vi "S2C_UNITHERM_Proc_Commands.vi"(7 "VI_Ref":refnum<vi>, 8 "Error In":errorcluster, 10 "Settings":T1, 11 "Q-Ref":refnum<queue>) -> (0 "Error Out":errorcluster, 2 "Stop?":bool, 3 "Response":variant)   [LabVIEW 2015]
uses:
  S2C_UNITHERM_Proc_Globals.vi
  _Shared/S2C_Shared_Proc_Globals.vi
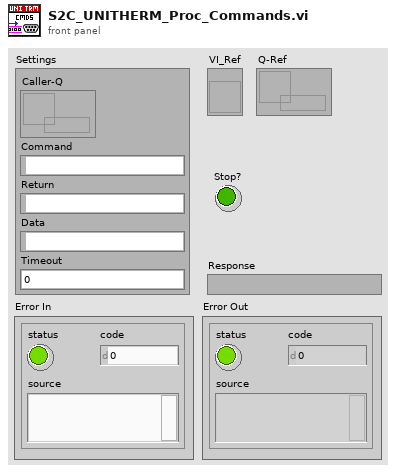
[diagram p1: front panel]
types:
  T1 = cluster{"Caller-Q":refnum<queue>, "Command":string, "Return":string, "Data":variant, "Timeout":dbl}
  T2 = enum16{"5190CR", "Fornax", "Omnia8257", "UniTherm"}
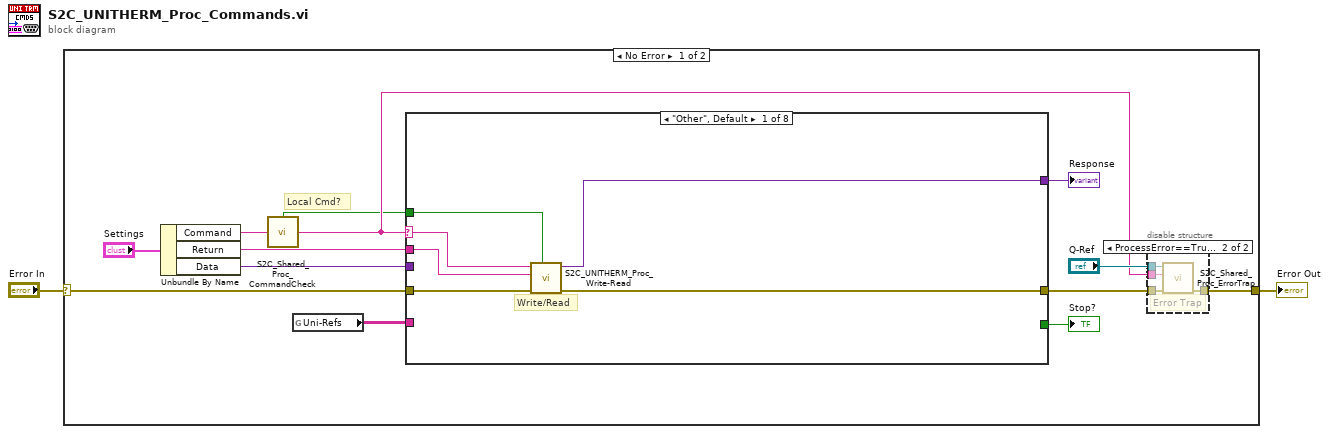
[diagram p0: block diagram]
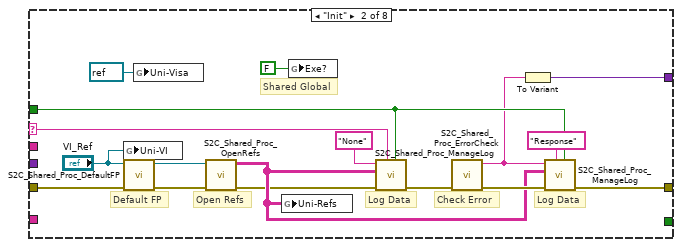
[diagram p3: hidden frame]
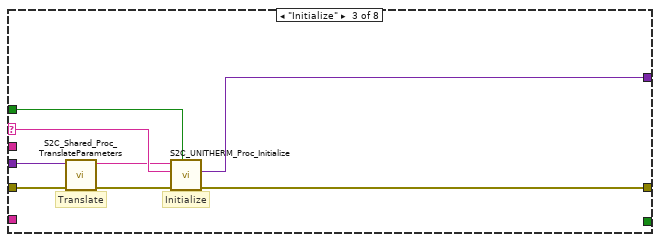
[diagram p4: hidden frame]
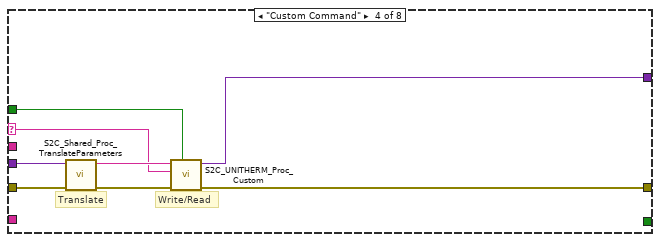
[diagram p5: hidden frame]
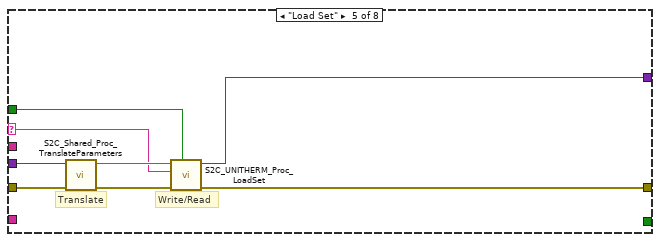
[diagram p6: hidden frame]
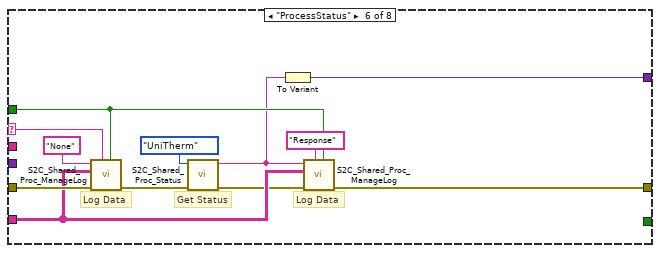
[diagram p7: hidden frame]
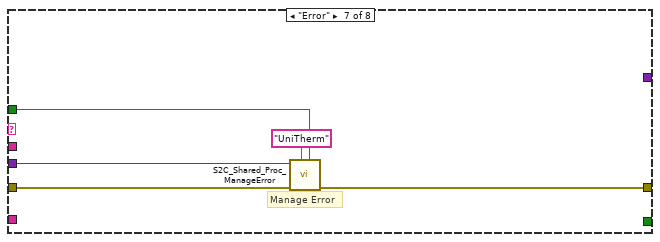
[diagram p8: hidden frame]
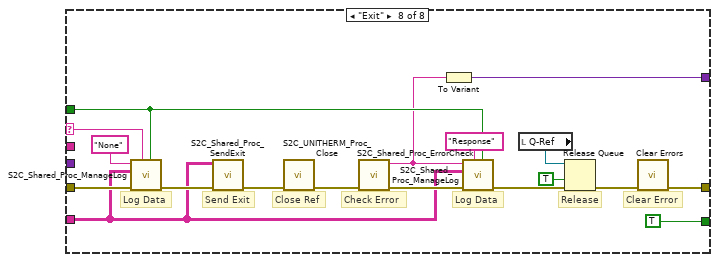
[diagram p9: hidden frame]
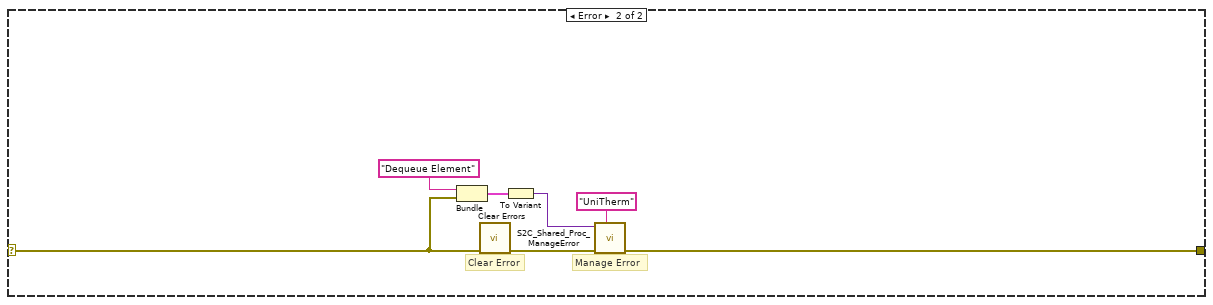
[diagram p10: hidden frame]
diagram:
  n1 = case shown="No Error" "Error In" {
    selector: "Error In" -> [w14 w106]
    tunnel: [w6 w108] -> w1
    frame No Error {
      # "Local Cmd?"
      n2 = Unbundle By Name("Settings") -> ("Command"=w5:string, "Return"=w10:string, "Data"=w15:variant)
      n3 = call "S2C_Shared_Proc_CommandCheck.vi"("Cmd In"=w5) -> ("Local?"=w3:bool, "Cmd Out"=w4:string)  [unwired: 13 in]
      n4 = global read "S2C_UNITHERM_Proc_Globals.vi" "Uni-Refs"() -> (w9:string[][])
      n5 = case shown="\"Other\", Default" w4 {
        selector: w4 -> [w22 w40 w47 w53 w61 w78 _ w99]
        tunnel: w14 -> [w24 w31 w51 w58 w66 w77 w83 w100]
        tunnel: w15 -> [_ _ w50 w57 w65 _ w80 _]
        tunnel: [w26 w43 w49 w59 w67 w74 w82 w85] -> w7
        tunnel: [w25 w37 w48 w56 w64 w75 _ w93] -> w12
        tunnel: [_ _ _ _ _ _ _ TRUE] -> w11
        tunnel: w10 -> [w21 _ _ _ _ _ _ _]
        tunnel: w3 -> [w23 w41 w44 w52 w60 w72 w81 w97]
        tunnel: w9 -> [_ _ _ _ _ w73 _ w90]
        frame "Other", Default {
          # "Write/Read"
          n6 = call "S2C_UNITHERM_Proc_Write-Read.vi"("Local?"=w23, "Error In"=w24, "Return"=w21, "Command"=w22) -> ("Error Out"=w26:errorcluster, "Response"=w25:variant)  [unwired: 6 in]
        }
        frame "Init" {
          # "Default FP"
          # "Shared Global"
          # "Check Error"
          # "Log Data"
          # "Open Refs"
          # "Log Data"
          n7 = global write "S2C_UNITHERM_Proc_Globals.vi" "Uni-VI"("VI_Ref") -> ()
          n8 = call "S2C_Shared_Proc_DefaultFP.vi"("Error In"=w31, "VI_Ref In"="VI_Ref") -> ("Error Out"=w28:errorcluster, "VI_Ref Out"=w29:refnum<vi>)  [unwired: 8 in]
          n9 = global write "S2C_UNITHERM_Proc_Globals.vi" "Uni-Visa"(refnum<visa-resource-name> refnum ("SerialRef")) -> ()
          n10 = call "S2C_Shared_Proc_OpenRefs.vi"("Error In"=w28, "VI_Ref"=w29) -> ("Error Out"=w32:errorcluster, "Refs"=w33:string[][])  [unwired: 8 in]
          n11 = global write "S2C_UNITHERM_Proc_Globals.vi" "Uni-Refs"(w33) -> ()
          n12 = global write "S2C_Shared_Proc_Globals.vi" "Exe?"(FALSE ("Exe?")) -> ()
          n13 = call "S2C_Shared_Proc_ManageLog.vi"("Local?"=w41, "Command"=w40, "Error In"=w32, "Refs"=w33, "Data In"="None") -> ("Error Out"=w35:errorcluster)  [unwired: 5 in, 1 out]
          n14 = call "S2C_Shared_Proc_ErrorCheck.vi"("Error In"=w35) -> ("Error Out"=w38:errorcluster, "Status"=w36:string)  [unwired: 9 in]
          n15 = To Variant(anything=w36) -> (Variant=w37:variant)
          n16 = call "S2C_Shared_Proc_ManageLog.vi"("Local?"=w41, "Command"="Response", "Error In"=w38, "Refs"=w33, "Data In"=w36) -> ("Error Out"=w43:errorcluster)  [unwired: 5 in, 1 out]
        }
        frame "Initialize" {
          # "Initialize"
          # "Translate"
          n17 = call "S2C_Shared_Proc_TranslateParameters.vi"("Error In"=w51, "Data"=w50) -> ("Error Out"=w46:errorcluster, "JSON Cluster"=w45:string)  [unwired: 8 in]
          n18 = call "S2C_UNITHERM_Proc_Initialize.vi"("Local?"=w44, "Error In"=w46, "Command"=w47, "JSON String"=w45) -> ("Error Out"=w49:errorcluster, "Response"=w48:variant)  [unwired: 6 in]
        }
        frame "Custom Command" {
          # "Write/Read"
          # "Translate"
          n19 = call "S2C_Shared_Proc_TranslateParameters.vi"("Error In"=w58, "Data"=w57) -> ("Error Out"=w55:errorcluster, "JSON Cluster"=w54:string)  [unwired: 8 in]
          n20 = call "S2C_UNITHERM_Proc_Custom.vi"("Local?"=w52, "Error In"=w55, "Command"=w53, "JSON String"=w54) -> ("Error Out"=w59:errorcluster, "Response"=w56:variant)  [unwired: 6 in]
        }
        frame "Load Set" {
          # "Write/Read"
          # "Translate"
          n21 = call "S2C_Shared_Proc_TranslateParameters.vi"("Error In"=w66, "Data"=w65) -> ("Error Out"=w63:errorcluster, "JSON Cluster"=w62:string)  [unwired: 8 in]
          n22 = call "S2C_UNITHERM_Proc_LoadSet.vi"("Local?"=w60, "Error In"=w63, "Command"=w61, "JSON String"=w62) -> ("Error Out"=w67:errorcluster, "Response"=w64:variant)  [unwired: 6 in]
        }
        frame "ProcessStatus" {
          # "Get Status"
          # "Log Data"
          # "Log Data"
          n23 = call "S2C_Shared_Proc_ManageLog.vi"("Local?"=w72, "Command"=w78, "Error In"=w77, "Refs"=w73, "Data In"="None") -> ("Error Out"=w71:errorcluster)  [unwired: 5 in, 1 out]
          n24 = call "S2C_Shared_Proc_Status.vi"("Error In"=w71, "Device"=T2."UniTherm") -> ("Error Out"=w69:errorcluster, "Response"=w68:string)  [unwired: 8 in]
          n25 = To Variant(anything=w68) -> (Variant=w75:variant)
          n26 = call "S2C_Shared_Proc_ManageLog.vi"("Local?"=w72, "Command"="Response", "Error In"=w69, "Refs"=w73, "Data In"=w68) -> ("Error Out"=w74:errorcluster)  [unwired: 5 in, 1 out]
        }
        frame "Error" {
          # "Manage Error"
          n27 = call "S2C_Shared_Proc_ManageError.vi"("Local?"=w81, "Process"="UniTherm", "Error In"=w83, "Data"=w80) -> ("Error Out"=w82:errorcluster)  [unwired: 7 in]
        }
        frame "Exit" {
          # "Clear Error"
          # "Release"
          # "Check Error"
          # "Send Exit"
          # "Log Data"
          # "Close Ref"
          # "Log Data"
          n28 = call "S2C_Shared_Proc_ManageLog.vi"("Local?"=w97, "Command"=w99, "Error In"=w100, "Refs"=w90, "Data In"="None") -> ("Error Out"=w91:errorcluster)  [unwired: 5 in, 1 out]
          n29 = call "S2C_Shared_Proc_SendExit.vi"("Error In"=w91, "Refs"=w90) -> ("Error Out"=w89:errorcluster)  [unwired: 9 in]
          n30 = call "S2C_UNITHERM_Proc_Close.vi"("Error In"=w89) -> ("Error Out"=w98:errorcluster)  [unwired: 10 in]
          n31 = call "S2C_Shared_Proc_ErrorCheck.vi"("Error In"=w98) -> ("Error Out"=w95:errorcluster, "Status"=w92:string)  [unwired: 9 in]
          n32 = To Variant(anything=w92) -> (Variant=w93:variant)
          n33 = call "S2C_Shared_Proc_ManageLog.vi"("Local?"=w97, "Command"="Response", "Error In"=w95, "Refs"=w90, "Data In"=w92) -> ("Error Out"=w94:errorcluster)  [unwired: 5 in, 1 out]
          n34 = local read "Q-Ref"() -> (w87:refnum<queue>)
          n35 = Release Queue(queue=w87, force destroy? (F)=TRUE, error in (no error)=w94) -> (error out=w88:errorcluster)  [unwired: 2 out]
          n36 = call <vilib>:"Clear Errors.vi"("error in (no error)"=w88) -> ("error out"=w85:errorcluster)  [unwired: 5 in, 1 out]
        }
      }
      "Response" <- w12
      "Stop?" <- w11
      n37 = disable-structure shown="ProcessError==True" {
        disable-tunnel: w7 -> [w16 w20]
        disable-tunnel: [w16 w19] -> w6
        disable-tunnel: w4 -> [_ w18]
        disable-tunnel: "Q-Ref" -> [_ w17]
        frame condition #0 (active) {
        }
        frame condition #1 {
          # "Error Trap"
          n38 = call "S2C_Shared_Proc_ErrorTrap.vi"("Error In"=w20, "Command"=w18, "Q-Ref"=w17) -> ("Error Out"=w19:errorcluster)  [unwired: 8 in]
        }
      }
    }
    frame Error {
      # "Clear Error"
      # "Manage Error"
      n39 = Bundle("Dequeue Element", "error IO"=w106) -> (w107:cluster{string, "error IO":errorcluster})  [unwired: 1 in]
      n40 = call <vilib>:"Clear Errors.vi"("error in (no error)"=w106) -> ("error out"=w103:errorcluster)  [unwired: 5 in, 1 out]
      n41 = To Variant(anything=w107) -> (Variant=w104:variant)
      n42 = call "S2C_Shared_Proc_ManageError.vi"("Process"="UniTherm", "Error In"=w103, "Data"=w104) -> ("Error Out"=w108:errorcluster)  [unwired: 8 in]
    }
  }
  "Error Out" <- w1
